vi "Update Transfer.vi"(8 "error in (no error)":errorcluster, 9 "data":string, 10 "Transfer":refnum<class "Transfer.lvclass">, 11 "UDP Transceiver in":refnum<class "UDP Transceiver.lvclass">) -> (0 "error out":errorcluster, 3 "UDP Transceiver out":refnum<class "UDP Transceiver.lvclass">)   [LabVIEW 2017, in "UDP Transceiver.lvlib" / "UDP Transceiver.lvclass"]
uses:
  UDP Transceiver.lvclass
  Builds/Data Sharing Framework/Current/Data Sharing Framework Core/DSF Core.lvlibp/Engine/Classes/Transfer/Transfer.lvclass
  UDP Size Mismatch Error.vi
  Builds/Data Sharing Framework/Current/Data Sharing Framework Core/DSF Core.lvlibp/Engine/Classes/Buffer/Buffer.lvclass
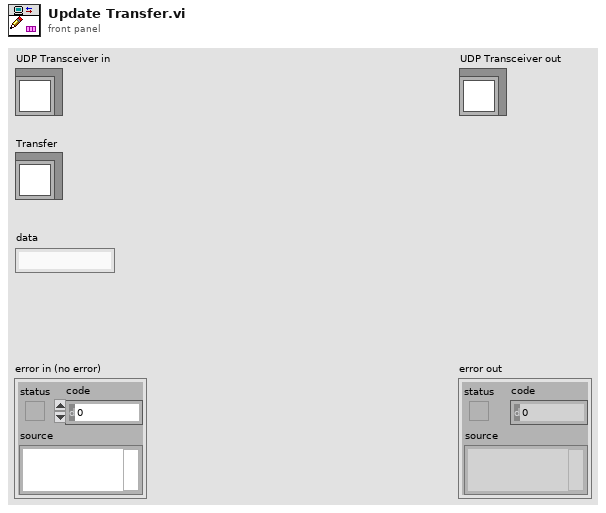
[diagram p1: front panel]
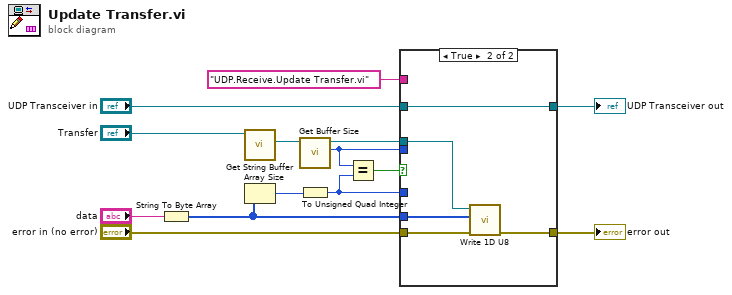
[diagram p0: block diagram]
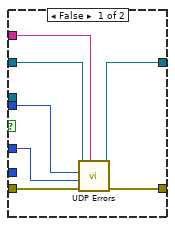
[diagram p2: hidden frame]
diagram:
  n1 = String To Byte Array(string="data") -> (unsigned byte array=w11:u8[])
  n2 = call "Get String Buffer.vi"("Transfer in"="Transfer") -> ("Buffer"=w14:refnum<class "Buffer.lvclass">)  [unwired: 9 in, 1 out]
  n3 = Array Size(array=w11) -> (size(s)=w13:i32)
  n4 = call "Get Buffer Size.vi"("Buffer in"=w14) -> ("buffer size"=w9:u64, "Buffer out"=w12:refnum<class "Buffer.lvclass">)  [unwired: 9 in]
  n5 = To Unsigned Quad Integer(1:w13) -> (0:w8:u64)
  n6 = Equal?(x=w9, y=w8) -> (x = y?=w10:bool)
  n7 = case shown="True" w10 {
    tunnel: w12 -> [_ w26]
    tunnel: "error in (no error)" -> [w21 w25]
    tunnel: [w20 w24] -> w4
    tunnel: w11 -> [_ w22]
    tunnel: "UDP Transceiver in" -> [w19 w23]
    tunnel: [w18 w23] -> w3
    tunnel: w9 -> [w16 _]
    tunnel: w8 -> [w17 _]
    tunnel: "UDP.Receive.Update Transfer.vi" ("source vi name") -> [w15 _]
    frame False {
      n8 = call-poly "UDP Errors.vi"("source vi name"=w15, "error in (no error)"=w21, "actual size"=w17, "expected size"=w16, "UDP in"=w19) -> ("error out"=w20:errorcluster, "UDP out"=w18:refnum<class "UDP Transceiver.lvclass">)  [unwired: 5 in]
    }
    frame True {
      n9 = call "Write 1D U8.vi"("error in (no error)"=w25, "buffer in"=w22, "Buffer in"=w26) -> ("error out"=w24:errorcluster)  [unwired: 5 in, 3 out]
    }
  }
  "error out" <- w4
  "UDP Transceiver out" <- w3
